vi "Main.vi"() -> ()   [LabVIEW 2018]
doc: "Cet exemple de projet Mesure continue est basé sur le modèle Gestionnaire de messages dans une file d'attente.\n\nLa boucle de gestion d'événements génère des messages en fonction des actions sur l'interface utilisateur.\n\nLa boucle de gestion de messages traite les messages générés par la boucle de gestion d'événements ou par d'autres messages. Il y a aussi des sous-VIs de boucle de gestion de messages d'acquisition et d'enregistrement, ainsi qu'une boucle de mise à jour du graphe déroulant."
uses:
  Acquisition/Acquisition.lvlib
  Logging/Logging.lvlib
  Settings/Settings.lvlib
  Acquisition/Signal Type.ctl
  Acquisition/Hardware Configuration.ctl
  Logging/Logging Configuration.ctl
  Settings/Settings.ctl
  support/User Event - Stop/User Event - Stop.lvlib
  controls/UI Data.ctl
  support/Message Queue/Message Queue.lvlib
  support/Message Queue/Enqueue Message (Single).vi
  controls/UI State.ctl
  <vilib>/ErrorRing/Error Ring.xnode
  Settings/Settings Dialog.vi
  support/Message Queue/Enqueue Message (Array).vi
  <vilib>/Utility/error.llb/Error Cluster From Error Code.vi
panel:
  in  "Panneaux":T1(tab)
  out "Therm 2":dbl(knob) scale=0.0..10.0
  out "Therm 1":dbl(knob) scale=0.0..10.0
  in  "Param status":bool
  out "Données":waveform(dbl)[](graph)
  out "État":string
  in  "Quitter":bool
  in  "Arrêter":bool
  in  "Démarrer":bool
  in  "Paramètres":bool
  # "MAPA Tech"
  # "TODO:\n\n- Valider l'enregistrement  du data\n- Faire sous-vi ordre 0\n- Faire sous-vi ordre 1"
  # "Changer tout cela pour des réservoir ou des vumètre ou jauge"
  # "MAPA Tech"
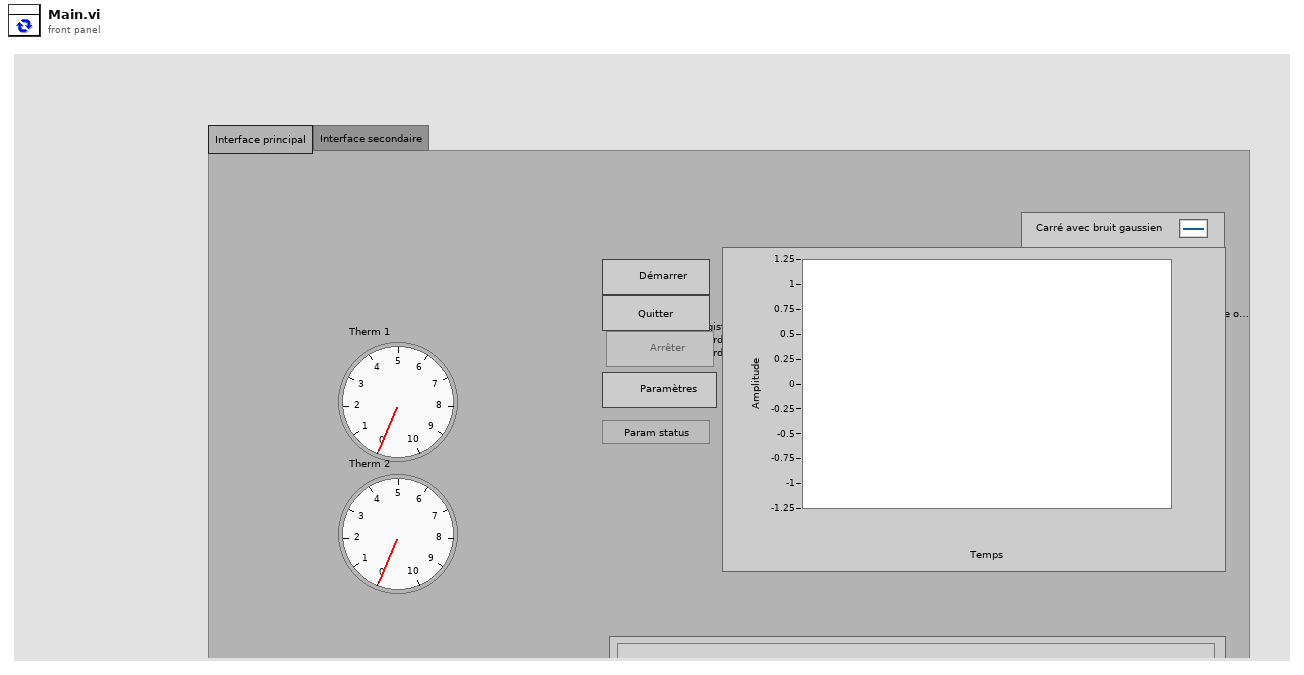
[diagram p1: front panel]
types:
  T1 = enum32{"Interface principal", "Interface secondaire"}
  T2 = typedef "UI State.ctl" = enum16{"Idle", "Acquiring and Logging", "Waiting for Exit", "Waiting for Exit (Acq Stopped)", "Waiting for Exit (Log Stopped)", "Waiting for Stop", "Waiting for Stop (Acq Stopped)", "Waiting for Stop (Log Stopped)"}
  T3 = typedef "UI Data.ctl" = cluster{"Réf. de Démarrer":refnum<vi>, "Réf. d'Arrêter":refnum<vi>, "Réf. de Paramètres":refnum<vi>, "Réf. de Quitter":refnum<vi>, "Réf. d'état":refnum<vi>, "Réf. de données":refnum<vi>, "Ref. Moyennage sélectionneur":refnum<vi>, "Ref. Param status":refnum<vi>}
  T4 = typedef "Settings.lvlib/Settings.ctl" = cluster{"Configuration du matériel":T5, "Configuration de l'enregistrement":T7}
  T5 = typedef "Acquisition.lvlib/Hardware Configuration.ctl" = cluster{"Refnum de matériel <À remplacer>":string, "Type de signal <À remplacer>":T6, "Choix de la longueur d'onde":dbl, "Nom du périphérique":tag, "Choix mode":bool}
  T6 = typedef "Acquisition.lvlib/Signal Type.ctl" = enum16{"Sine Wave", "Square with Noise", "Signal triangulaire", "Simulation DAQ"}
  T7 = typedef "Logging.lvlib/Logging Configuration.ctl" = cluster{"Chemin de base du fichier journal":path, "Référence de fichier TDMS":refnum<k34>}
  T8 = cluster{"état":bool, "code":i32, "source":string}
  T9 = typedef "Message Queue.lvlib/All Message Queues.ctl" = cluster{"IU":refnum<queue>, "Acquisition":refnum<queue>, "Enregistrement":refnum<queue>}
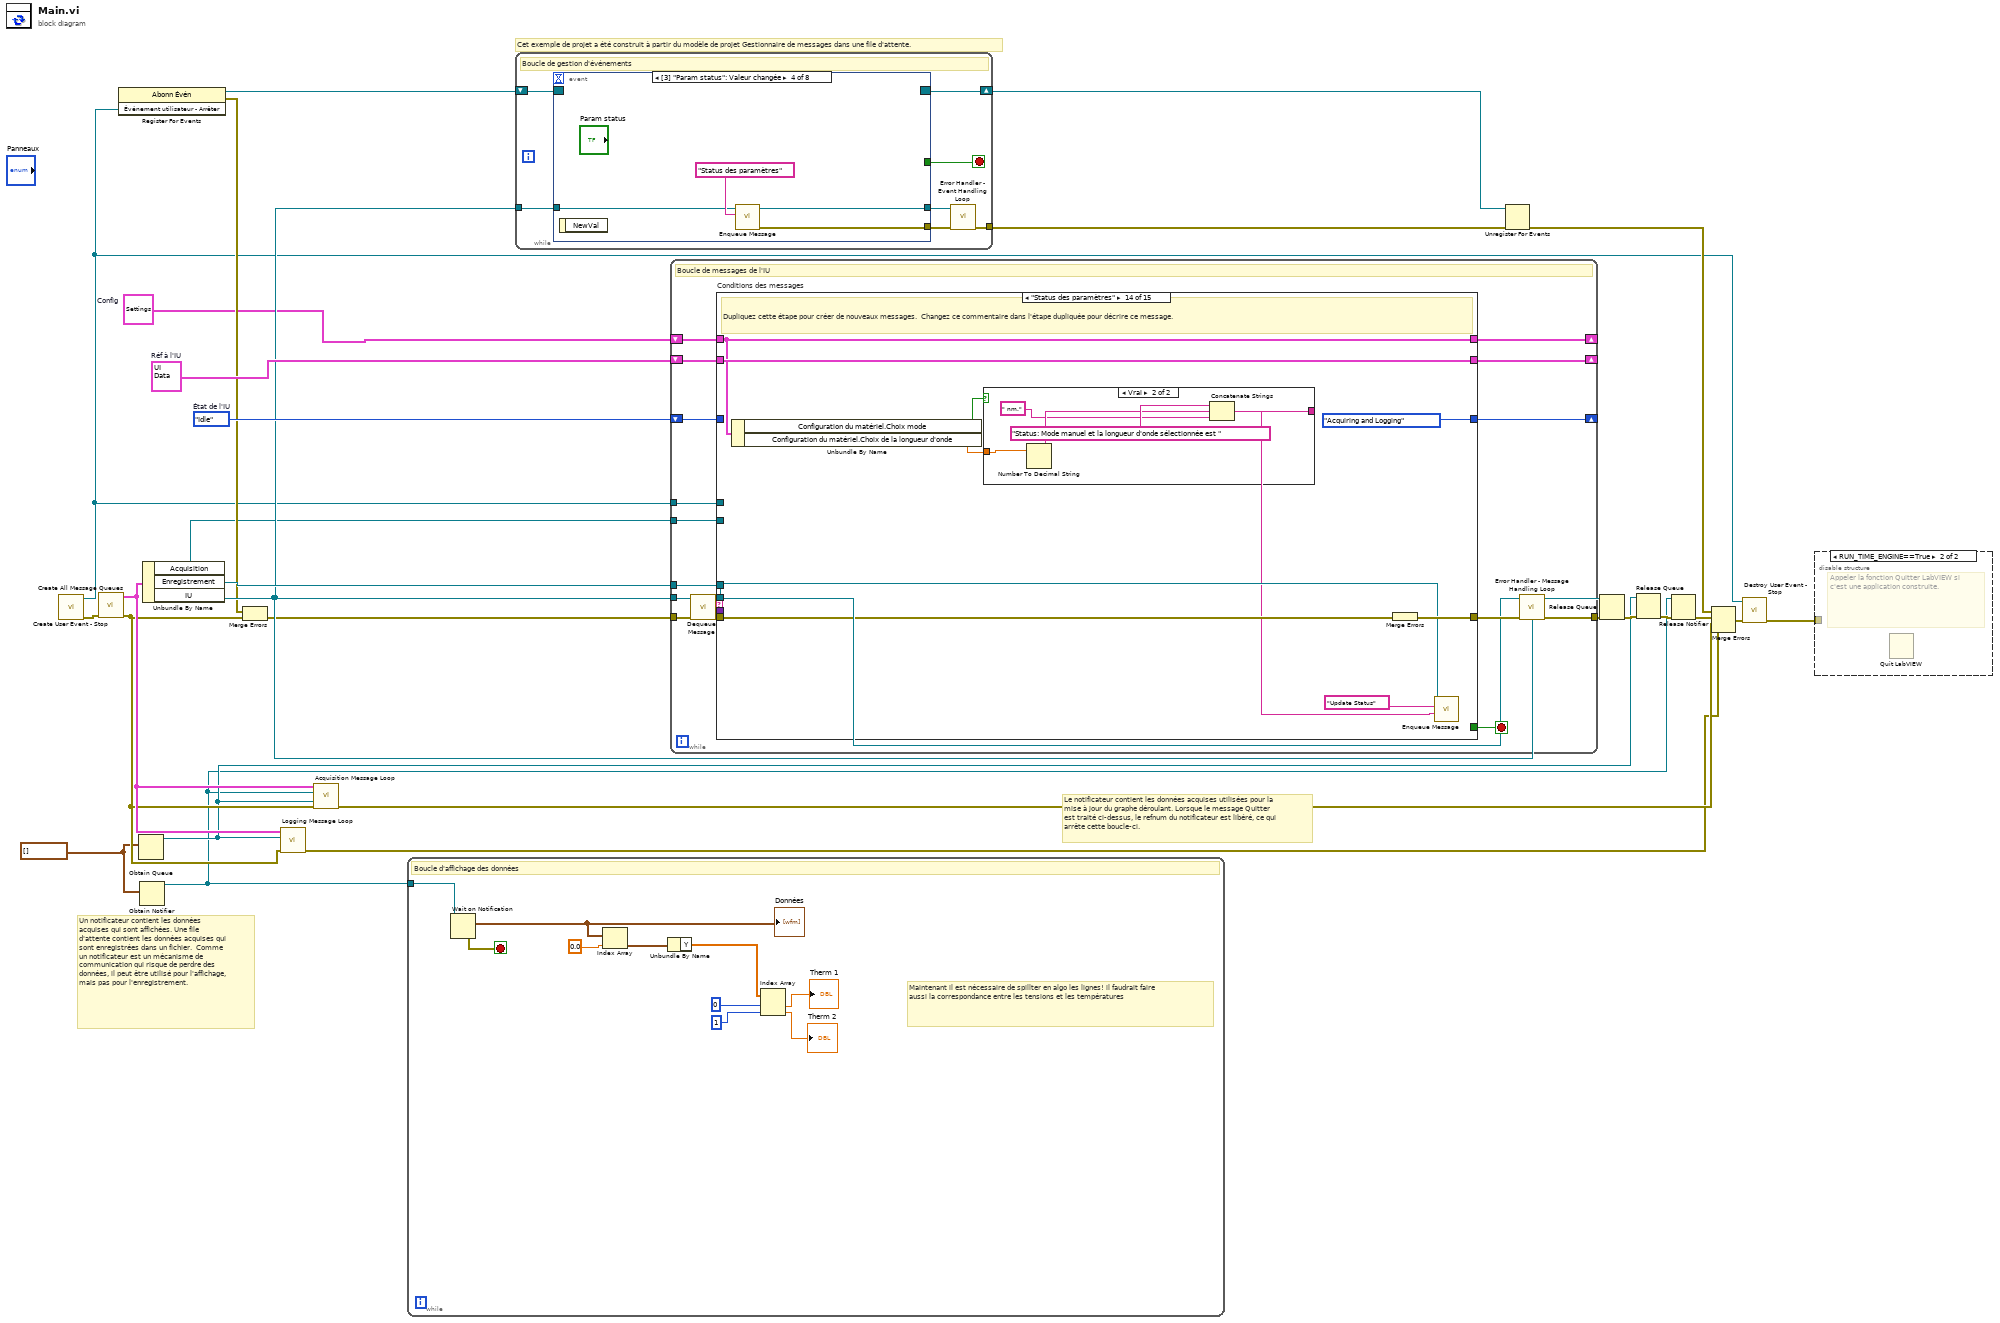
[diagram p0: block diagram]
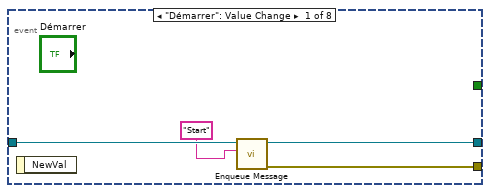
[diagram p3: hidden frame]
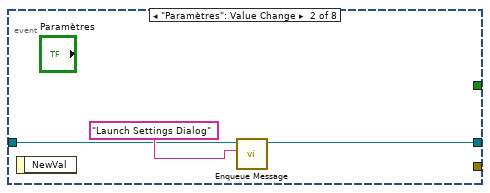
[diagram p4: hidden frame]
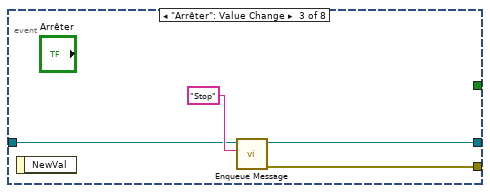
[diagram p5: hidden frame]
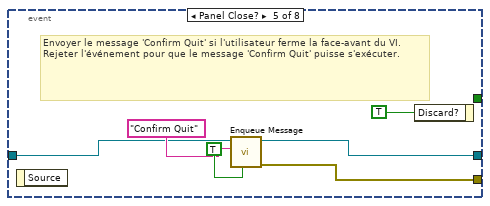
[diagram p6: hidden frame]
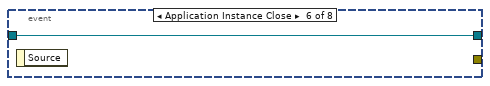
[diagram p7: hidden frame]
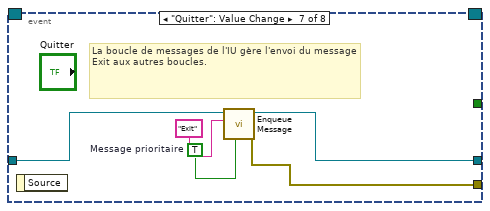
[diagram p8: hidden frame]
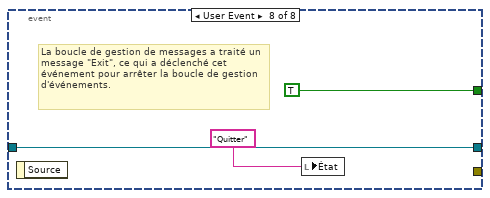
[diagram p9: hidden frame]
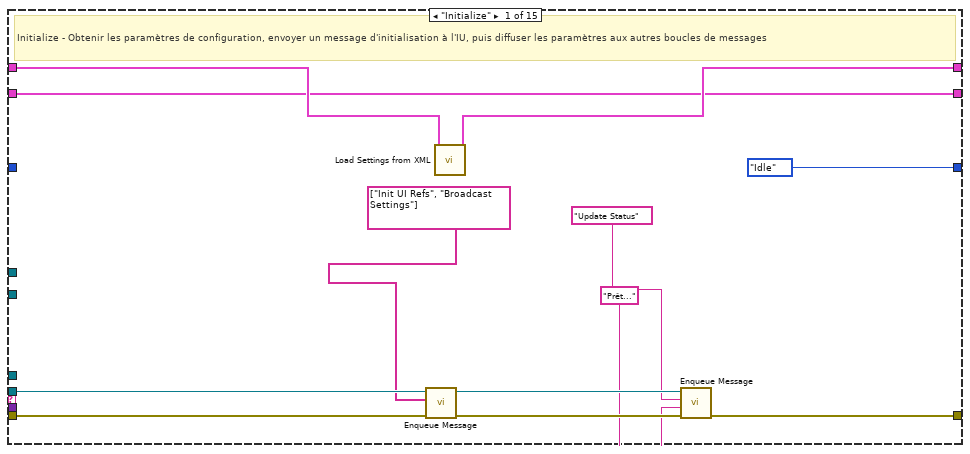
[diagram p10: hidden frame]
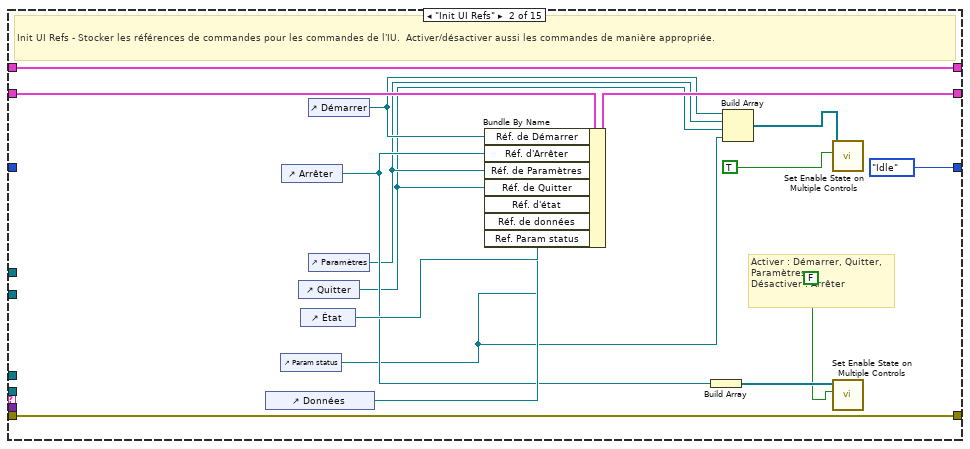
[diagram p11: hidden frame]
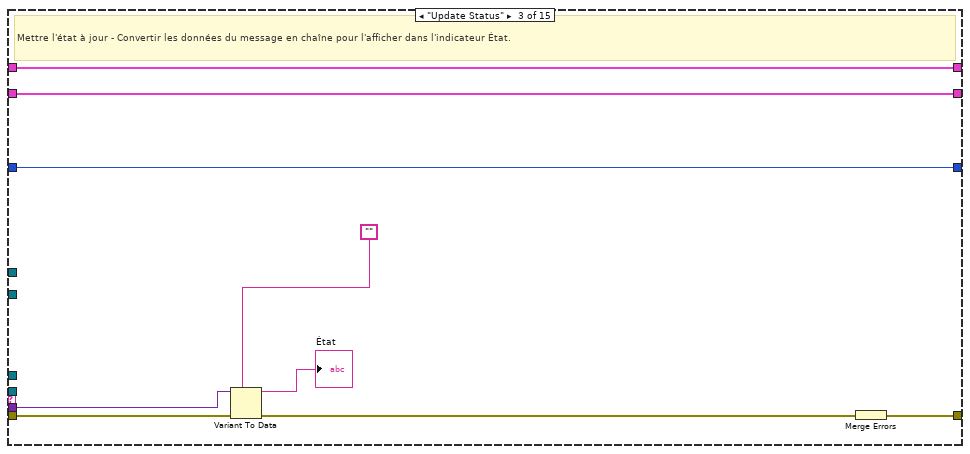
[diagram p12: hidden frame]
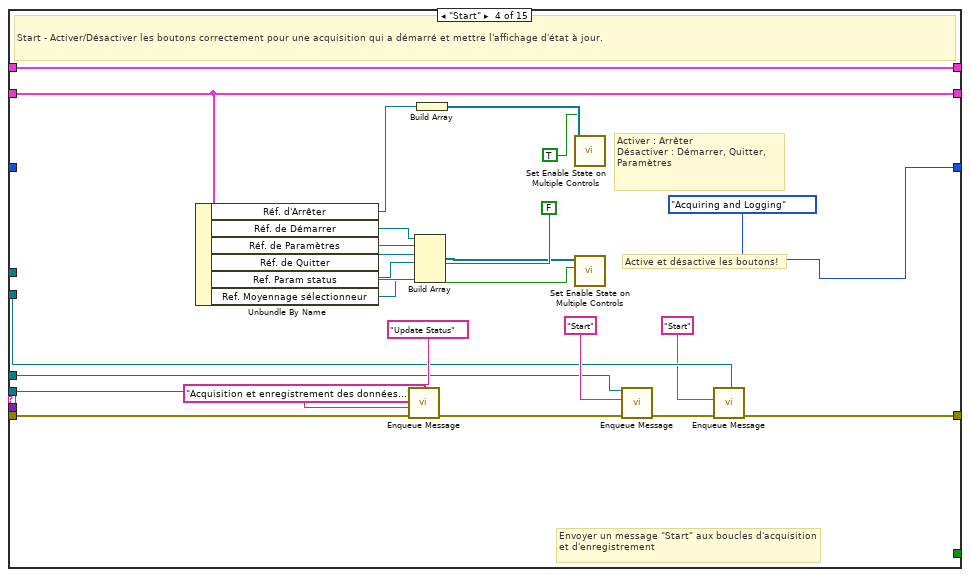
[diagram p13: hidden frame]
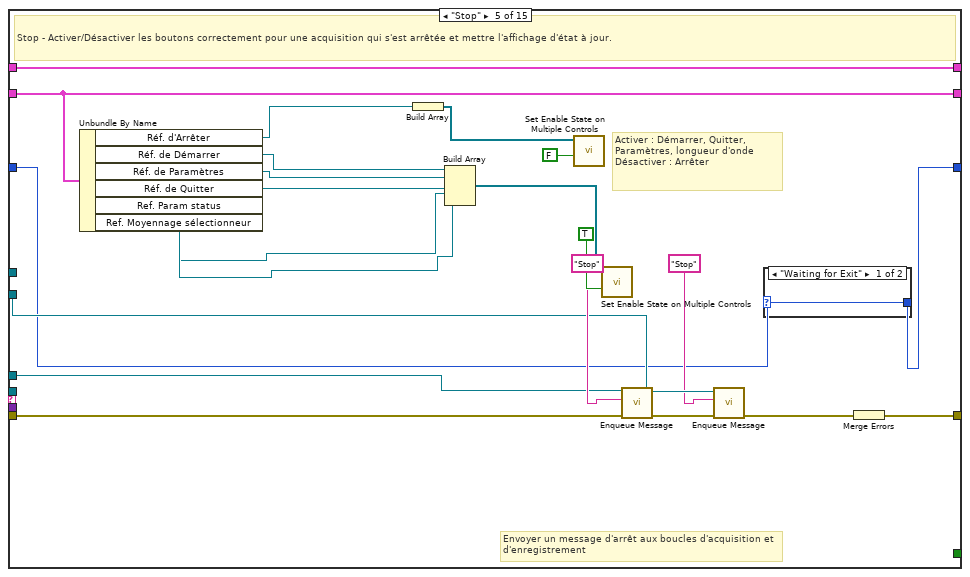
[diagram p14: hidden frame]
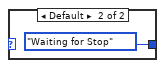
[diagram p15: hidden frame]
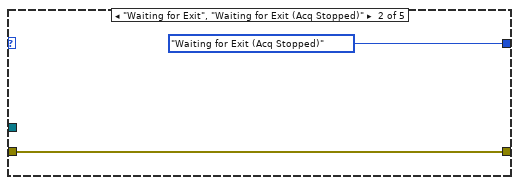
[diagram p17: hidden frame]
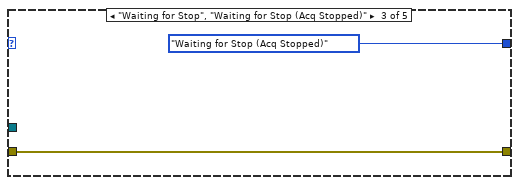
[diagram p18: hidden frame]
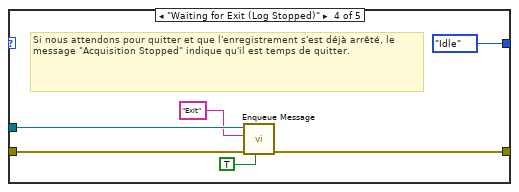
[diagram p19: hidden frame]
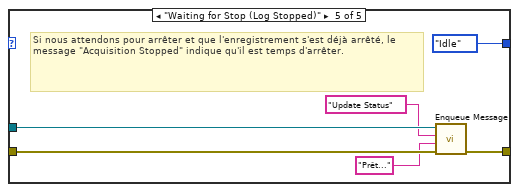
[diagram p20: hidden frame]
diagram:
  w16 = UI_State."Idle"  # État de l'IU
  w4 = waveform(dbl)[] []
  w18 = T3 {"Réf. de Démarrer"=refnum, "Réf. d'Arrêter"=refnum, "Réf. de Paramètres"=refnum, "Réf. de Quitter"=refnum, "Réf. d'état"=refnum, "Réf. de données"=refnum, "Ref. Moyennage sélectionneur"=refnum, "Ref. Param status"=refnum}  # Réf à l'IU
  w1 = T4 {"Configuration du matériel"={"Refnum de matériel <À remplacer>"="", "Type de signal <À remplacer>"=enum."Simulation DAQ", "Choix de la longueur d'onde"=500.0, "Nom du périphérique"="Dev1", "Choix mode"=FALSE}, "Configuration de l'enregistrement"={"Chemin de base du fichier journal"=path "", "Référence de fichier TDMS"=refnum}}  # Config
  # "Cet exemple de projet a été construit à partir du modèle de projet Gestionnaire de messages dans une file d'attente."
  # "Un notificateur contient les données acquises qui sont affichées. Une file d'attente contient les données acquises qui sont enregistrées dans un fichier.  Comme un notificateur est un mécanisme de communication qui risque de perdre des données, il peut être utilisé pour l'affichage, mais pas pour l'enregistrement."
  # "Le notificateur contient les données acquises utilisées pour la mise à jour du graphe déroulant. Lorsque le message Quitter est traité ci-dessus, le refnum du notificateur est libéré, ce qui arrête cette boucle-ci."
  n1 = call "Create User Event - Stop.vi"() -> ("error out"=w24:T8, "Événement utilisateur - Arrêter"=w5:refnum<user-event>)  [unwired: 10 in]
  n2 = call "Create All Message Queues.vi"("error in (no error)"=w24) -> ("error out"=w21:T8, "Files d'attente de messages en sortie"=w23:T9)  [unwired: 9 in]
  n3 = register-events(w5) -> (reference out=w9:refnum<event-registration>, error out=w7:errorcluster)  [unwired: 2 in]
  n4 = Obtain Queue(element data type=w4) -> (queue out=w3:refnum<queue>)  [unwired: 4 in, 2 out]
  n5 = Obtain Notifier(notification data type=w4) -> (notifier out=w2:refnum<notifier>)  [unwired: 3 in, 2 out]
  n6 = Unbundle By Name(w23) -> ("Acquisition"=w6:refnum<queue>, "Enregistrement"=w17:refnum<queue>, "IU"=w14:refnum<queue>)
  n7 = Merge Errors(w7, w21) -> (w8:errorcluster)
  n8 = call "Logging Message Loop.vi"("error in (no error)"=w21, "File d'attente de données"=w3, "Files d'attente de messages"=w23) -> ("error out"=w22:T8)  [unwired: 8 in]
  n9 = call "Acquisition Message Loop.vi"("Files d'attente de messages"=w23, "Notificateur de données"=w2, "File d'attente de données"=w3, "error in (no error)"=w21) -> ("error out"=w25:T8)  [unwired: 11 in]
  n10 = while "Data Display Loop" {
    tunnel: w2 -> [w36]
    stop <- w37 stop-if-true
    # "Maintenant il est nécessaire de spillter en algo les lignes! il faudrait faire aussi la correspondance entre les tensions et les températures"
    # "Boucle d'affichage des données"
    n11 = Wait on Notification(notifier=w36) -> (notification=w34:waveform(dbl)[], error out=w37:errorcluster)  [unwired: 3 in, 2 out]
    "Données" <- w34
    n12 = Index Array(array=w34, index=0.0) -> (element=w33:waveform(dbl))
    n13 = Unbundle By Name(w33) -> ("Y"=w32:dbl[])
    n14 = Index Array(array=w32, index #1=0, index #2=1) -> (element #1=→"Therm 1":dbl, element #2=→"Therm 2":dbl)
  }
  n15 = while {
    tunnel: w14 -> [w43]
    tunnel: [w40] -> w26
    shift-right: [w42] -> w19
    shift-left: w9 -> [w44]
    stop <- w41 stop-if-true
    # "Boucle de gestion d'événements"
    n16 = event shown="[3] \"Param status\": Valeur changée" {
      selector: w44 -> [_ _ _ _ _ _ _ _]
      dyn-events: [_ _ _ _ _ _ _ _] -> w42
      timeout: _ -> [_ _ _ _ _ _ _ _]
      tunnel: [_ _ _ _ _ _ _ TRUE ("Discard?")] -> w41
      tunnel: w43 -> [w48 w50 w54 w58 w63 w66 w68 w72]
      tunnel: [w46 _ w53 w57 w61 _ w71 _] -> w39
      tunnel: [w45 w49 w52 w56 w62 w66 w67 w72] -> w38
      event "Démarrer": Value Change {
        n17 = event-data() -> ()  [unwired: 1 in, 1 out]
        n18 = call-poly "Enqueue Message.vi"("Message"="Start", "File d'attente de messages"=w48) -> ("error out"=w46:T8, "File d'attente de message dup."=w45:refnum<queue>)  [unwired: 8 in]
      }
      event "Paramètres": Value Change {
        n19 = event-data() -> ()  [unwired: 1 in, 1 out]
        n20 = call-poly "Enqueue Message.vi"("Message"="Launch Settings Dialog", "File d'attente de messages"=w50) -> ("File d'attente de message dup."=w49:refnum<queue>)  [unwired: 8 in, 1 out]
      }
      event "Arrêter": Value Change {
        n21 = event-data() -> ()  [unwired: 1 in, 1 out]
        n22 = call-poly "Enqueue Message.vi"("Message"="Stop", "File d'attente de messages"=w54) -> ("error out"=w53:T8, "File d'attente de message dup."=w52:refnum<queue>)  [unwired: 8 in]
      }
      event "Param status": Value Change {
        n23 = event-data() -> ()  [unwired: 1 in, 1 out]
        n24 = call-poly "Enqueue Message.vi"("Message"="Status des paramètres", "File d'attente de messages"=w58) -> ("error out"=w57:T8, "File d'attente de message dup."=w56:refnum<queue>)  [unwired: 8 in]
      }
      event Panel Close? {
        # "Envoyer le message 'Confirm Quit' si l'utilisateur ferme la face-avant du VI. Rejeter l'événement pour que le message 'Confirm Quit' puisse s'exécuter."
        n25 = event-data() -> ()  [unwired: 1 in, 1 out]
        n26 = call-poly "Enqueue Message.vi"("Message prioritaire ? (F)"=TRUE ("Priority Message? (F)"), "Message"="Confirm Quit", "File d'attente de messages"=w63) -> ("error out"=w61:T8, "File d'attente de message dup."=w62:refnum<queue>)  [unwired: 7 in]
        n27 = event-data ("Event Filter Node")("Discard?"=TRUE) -> ()  [unwired: 1 in, 1 out]
      }
      event Application Instance Close {
        n28 = event-data() -> ()  [unwired: 1 in, 1 out]
      }
      event "Quitter": Value Change {
        w69 = TRUE  # Message prioritaire
        # "La boucle de messages de l'IU gère l'envoi du message Exit aux autres boucles."
        n29 = event-data() -> ()  [unwired: 1 in, 1 out]
        n30 = call-poly "Enqueue Message.vi"("Message prioritaire ? (F)"=w69, "Message"="Exit", "File d'attente de messages"=w68) -> ("error out"=w71:T8, "File d'attente de message dup."=w67:refnum<queue>)  [unwired: 7 in]
      }
      event User Event {
        # "La boucle de gestion de messages a traité un message \"Exit\", ce qui a déclenché cet événement pour arrêter la boucle de gestion d'événements."
        n31 = event-data() -> ()  [unwired: 1 in, 1 out]
        n32 = local write "État"("Quitter" ("Exit String")) -> ()
      }
    }
    n33 = call "Error Handler - Event Handling Loop.vi"("error in (no error)"=w39, "File d'attente de messages"=w38) -> ("erreur en entrée dup."=w40:T8)  [unwired: 8 in, 1 out]
  }
  n34 = while {
    tunnel: w14 -> [w86]
    tunnel: w5 -> [w91]
    shift-right: [w85] -> _
    shift-left: w1 -> [w84]
    shift-right: [w82] -> _
    shift-left: w18 -> [w83]
    tunnel: w6 -> [w81]
    tunnel: w17 -> [w80]
    shift-right: [w75] -> _
    shift-left: w16 -> [w76]
    tunnel: w8 -> [w90]
    tunnel: [w79] -> w27
    stop <- w92 stop-if-true
    # "Boucle de messages de l'IU"
    n35 = call "Dequeue Message.vi"("error in (no error)"=w90, "File d'attente de messages"=w86) -> ("error out"=w89:T8, "Données de message"=w87:variant, "Message"=w88:string, "File d'attente de message dup."=w77:refnum<queue>)  [unwired: 6 in]
    n36 = case "Conditions des messages" shown="\"Status des paramètres\"" w88 {
      selector: w88 -> [_ _ _ _ _ _ _ _ _ _ _ _ _ _ w330]
      tunnel: w77 -> [w96 _ _ w153 _ w180 w205 _ w245 _ w266 _ _ w317 _]
      tunnel: w89 -> [w95 w120 w128 w152 w174 w181 w206 w233 w247 w254 w265 w294 w311 w321 _]
      tunnel: [w100 w120 w129 w139 w175 w178 w203 w239 w240 w257 w264 w304 w310 w320 w329] -> w78
      tunnel: [_ _ _ _ _ _ _ _ _ _ _ TRUE _ _ _] -> w92
      tunnel: w87 -> [_ _ w127 _ _ _ _ _ _ w258 _ w292 _ _ _]
      tunnel: w91 -> [_ _ _ _ _ _ _ _ _ _ _ w305 _ _ _]
      tunnel: [w103 w119 w123 w151 w173 w184 w209 w237 w244 w262 w269 w303 w309 w315 w333] -> w85
      tunnel: w84 -> [w104 w119 w123 w151 w173 w184 w209 w237 w248 w262 w269 w303 w309 w315 w333]
      tunnel: w83 -> [w97 w118 w122 w148 w172 w183 w208 w232 w242 w261 w268 w302 w308 w319 w332]
      tunnel: [w97 w115 w122 w148 w172 w183 w208 w232 w242 w261 w268 w302 w308 w319 w332] -> w82
      tunnel: w81 -> [_ _ _ w138 w165 _ _ w231 _ _ _ w301 _ _ _]
      tunnel: w80 -> [_ _ _ w141 w168 _ _ w228 _ _ _ w300 _ _ _]
      tunnel: w76 -> [_ _ w121 _ w162 w182 w207 w230 w241 w256 w267 _ w307 _ w331]
      tunnel: [UI_State."Idle" ("UI State") UI_State."Idle" ("UI State") w121 UI_State."Acquiring and Logging" ("UI State") w163 w179 w204 w230 w241 w256 w263 UI_State."Idle" ("UI State") w307 UI_State."Acquiring and Logging" ("UI State") w331] -> w75
      frame "Initialize" {
        # "Initialize - Obtenir les paramètres de configuration, envoyer un message d'initialisation à l'IU, puis diffuser les paramètres aux autres boucles de messages"
        n37 = call-poly "Enqueue Message.vi"("error in (no error)"=w95, "Tableau de messages"=string[] ["Init UI Refs", "Broadcast Settings"], "File d'attente de messages"=w96) -> ("error out"=w102:T8, "File d'attente de message dup."=w101:refnum<queue>)  [unwired: 7 in]
        n38 = call "Load Settings from XML.vi"("Paramètres en entrée"=w104) -> ("Paramètres en sortie"=w103:T4)  [unwired: 9 in, 1 out]
        n39 = call-poly "Enqueue Message.vi"("error in (no error)"=w102, "Données de message"="Prêt..." ("Ready..."), "Message"="Update Status", "File d'attente de messages"=w101) -> ("error out"=w100:T8)  [unwired: 6 in, 1 out]
      }
      frame "Init UI Refs" {
        # "Activer : Démarrer, Quitter, Paramètres\nDésactiver : Arrêter"
        # "Init UI Refs - Stocker les références de commandes pour les commandes de l'IU.  Activer/désactiver aussi les commandes de manière appropriée."
        n40 = control-ref of="Données"() -> (w116:refnum<vi>)
        n41 = control-ref of="Param status"() -> (w105:refnum<vi>)
        n42 = control-ref of="Arrêter"() -> (w110:refnum<vi>)
        n43 = control-ref of="Quitter"() -> (w107:refnum<vi>)
        n44 = control-ref of="État"() -> (w117:refnum<vi>)
        n45 = control-ref of="Démarrer"() -> (w109:refnum<vi>)
        n46 = control-ref of="Paramètres"() -> (w108:refnum<vi>)
        n47 = Bundle By Name(cluster=w118, "Réf. de Démarrer"=w109, "Réf. d'Arrêter"=w110, "Réf. de Paramètres"=w108, "Réf. de Quitter"=w107, "Réf. d'état"=w117, "Réf. de données"=w116, "Ref. Param status"=w105) -> (w115:T3)
        n48 = Build Array(w110) -> (w112:refnum<vi>[])
        n49 = Build Array(w109, w108, w107, w105) -> (w113:refnum<vi>[])
        n50 = call "Set Enable State on Multiple Controls.vi"("Activé ?"=TRUE ("Enable?"), "Commandes"=w113) -> ()  [unwired: 10 in]
        n51 = call "Set Enable State on Multiple Controls.vi"("Activé ?"=FALSE ("Enable?"), "Commandes"=w112) -> ()  [unwired: 10 in]
      }
      frame "Update Status" {
        # "Mettre l'état à jour - Convertir les données du message en chaîne pour l'afficher dans l'indicateur État."
        n52 = Variant To Data(error in=w128, type="" ("Empty String Constant"), Variant=w127) -> (data=→"État":string, error out=w125:errorcluster)
        n53 = Merge Errors(w125) -> (w129:errorcluster)
      }
      frame "Start" {
        # "Active et désactive les boutons!"
        # "Envoyer un message \"Start\" aux boucles d'acquisition et d'enregistrement"
        # "Activer : Arrêter\nDésactiver : Démarrer, Quitter, Paramètres"
        # "Start - Activer/Désactiver les boutons correctement pour une acquisition qui a démarré et mettre l'affichage d'état à jour."
        n54 = Unbundle By Name(w148) -> ("Réf. d'Arrêter"=w130:refnum<vi>, "Réf. de Démarrer"=w131:refnum<vi>, "Réf. de Paramètres"=w132:refnum<vi>, "Réf. de Quitter"=w135:refnum<vi>, "Ref. Param status"=w134:refnum<vi>, "Ref. Moyennage sélectionneur"=w133:refnum<vi>)
        n55 = call-poly "Enqueue Message.vi"("error in (no error)"=w152, "Données de message"="Acquisition et enregistrement des données..." ("Acquiring and Logging..."), "Message"="Update Status", "File d'attente de messages"=w153) -> ("error out"=w143:T8)  [unwired: 6 in, 1 out]
        n56 = Build Array(w131, w132, w132, w135, w134, w133) -> (w146:refnum<vi>[])
        n57 = Build Array(w130) -> (w145:refnum<vi>[])
        n58 = call "Set Enable State on Multiple Controls.vi"("Activé ?"=TRUE ("Enable?"), "Commandes"=w145) -> ()  [unwired: 10 in]
        n59 = call "Set Enable State on Multiple Controls.vi"("Activé ?"=FALSE ("Enable?"), "Commandes"=w146) -> ()  [unwired: 10 in]
        n60 = call-poly "Enqueue Message.vi"("error in (no error)"=w143, "Message"="Start", "File d'attente de messages"=w141) -> ("error out"=w140:T8)  [unwired: 7 in, 1 out]
        n61 = call-poly "Enqueue Message.vi"("error in (no error)"=w140, "Message"="Start", "File d'attente de messages"=w138) -> ("error out"=w139:T8)  [unwired: 7 in, 1 out]
      }
      frame "Stop" {
        # "Envoyer un message d'arrêt aux boucles d'acquisition et d'enregistrement"
        # "Activer : Démarrer, Quitter, Paramètres, longueur d'onde\nDésactiver : Arrêter"
        # "Stop - Activer/Désactiver les boutons correctement pour une acquisition qui s'est arrêtée et mettre l'affichage d'état à jour."
        n62 = Unbundle By Name(w172) -> ("Réf. d'Arrêter"=w154:refnum<vi>, "Réf. de Démarrer"=w155:refnum<vi>, "Réf. de Paramètres"=w156:refnum<vi>, "Réf. de Quitter"=w157:refnum<vi>, "Ref. Param status"=w158:refnum<vi>, "Ref. Moyennage sélectionneur"=w159:refnum<vi>)
        n63 = Build Array(w154) -> (w160:refnum<vi>[])
        n64 = Build Array(w155, w156, w157, w158, w159) -> (w161:refnum<vi>[])
        n65 = call "Set Enable State on Multiple Controls.vi"("Activé ?"=FALSE ("Enable?"), "Commandes"=w160) -> ()  [unwired: 10 in]
        n66 = call "Set Enable State on Multiple Controls.vi"("Activé ?"=TRUE ("Enable?"), "Commandes"=w161) -> ()  [unwired: 10 in]
        n67 = call-poly "Enqueue Message.vi"("error in (no error)"=w174, "Message"="Stop", "File d'attente de messages"=w168) -> ("error out"=w167:T8)  [unwired: 7 in, 1 out]
        n68 = call-poly "Enqueue Message.vi"("error in (no error)"=w167, "Message"="Stop", "File d'attente de messages"=w165) -> ("error out"=w166:T8)  [unwired: 7 in, 1 out]
        n69 = case shown="\"Waiting for Exit\"" w162 {
          selector: w162 -> [w176 _]
          tunnel: [w176 UI_State."Waiting for Stop" ("UI State")] -> w163
          frame "Waiting for Exit" {
          }
          frame Default {
          }
        }
        n70 = Merge Errors(w166) -> (w175:errorcluster)
      }
      frame "Acquisition Stopped" {
        # "Logique déterminant quelle action entreprendre quand l'acquisition s'est arrêtée."
        n71 = case shown="Par défaut" w182 {
          selector: w182 -> [w186 _ _ _ _]
          tunnel: w181 -> [w185 w188 w190 w196 w202]
          tunnel: w180 -> [_ _ _ w194 w199]
          tunnel: [w186 UI_State."Waiting for Exit (Acq Stopped)" ("UI State") UI_State."Waiting for Stop (Acq Stopped)" ("UI State") UI_State."Idle" ("UI State") UI_State."Idle" ("UI State")] -> w179
          tunnel: [w185 w188 w190 w195 w200] -> w178
          frame Default {
          }
          frame "Waiting for Exit", "Waiting for Exit (Acq Stopped)" {
          }
          frame "Waiting for Stop", "Waiting for Stop (Acq Stopped)" {
          }
          frame "Waiting for Exit (Log Stopped)" {
            # "Si nous attendons pour quitter et que l'enregistrement s'est déjà arrêté, le message \"Acquisition Stopped\" indique qu'il est temps de quitter."
            n72 = call-poly "Enqueue Message.vi"("Message prioritaire ? (F)"=TRUE ("Priority Message? (F)"), "error in (no error)"=w196, "Message"="Exit", "File d'attente de messages"=w194) -> ("error out"=w195:T8)  [unwired: 6 in, 1 out]
          }
          frame "Waiting for Stop (Log Stopped)" {
            # "Si nous attendons pour arrêter et que l'enregistrement s'est déjà arrêté, le message \"Acquisition Stopped\" indique qu'il est temps d'arrêter."
            n73 = call-poly "Enqueue Message.vi"("error in (no error)"=w202, "Données de message"="Prêt..." ("Ready..."), "Message"="Update Status", "File d'attente de messages"=w199) -> ("error out"=w200:T8)  [unwired: 6 in, 1 out]
          }
        }
      }
      frame "Logging Stopped" {
        # "Logique déterminant quelle action entreprendre quand l'enregistrement s'est arrêté."
        n74 = case shown="\"Waiting for Stop (Acq Stopped)\"" w207 {
          selector: w207 -> [w211 _ _ _ _]
          tunnel: w206 -> [w210 w213 w215 w221 w224]
          tunnel: w205 -> [_ _ _ w219 w223]
          tunnel: [w211 UI_State."Waiting for Exit (Log Stopped)" ("UI State") UI_State."Waiting for Stop (Log Stopped)" ("UI State") UI_State."Idle" ("UI State") UI_State."Idle" ("UI State")] -> w204
          tunnel: [w210 w213 w215 w220 w222] -> w203
          frame Default {
          }
          frame "Waiting for Exit", "Waiting for Exit (Log Stopped)" {
          }
          frame "Waiting for Stop", "Waiting for Stop (Log Stopped)" {
          }
          frame "Waiting for Exit (Acq Stopped)" {
            # "Si nous attendons pour quitter et que l'acquisition s'est déjà arrêtée, le message \"Logging Stopped\" indique qu'il est temps de quitter."
            n75 = call-poly "Enqueue Message.vi"("Message prioritaire ? (F)"=TRUE ("Priority Message? (F)"), "error in (no error)"=w221, "Message"="Exit", "File d'attente de messages"=w219) -> ("error out"=w220:T8)  [unwired: 6 in, 1 out]
          }
          frame "Waiting for Stop (Acq Stopped)" {
            # "Si nous attendons pour arrêter et que l'acquisition s'est déjà arrêtée, le message \"Logging Stopped\" indique qu'il est temps d'arrêter."
            n76 = call-poly "Enqueue Message.vi"("error in (no error)"=w224, "Données de message"="Prêt..." ("Ready..."), "Message"="Update Status", "File d'attente de messages"=w223) -> ("error out"=w222:T8)  [unwired: 6 in, 1 out]
          }
        }
      }
      frame "Broadcast settings" {
        w229 = "Update Settings" ("Message")
        # "Broadcast settings - Envoyer le message 'Update Settings' aux boucles de messages d'enregistrement et d'acquisition."
        n77 = Unbundle By Name(w237) -> ("Configuration du matériel"=w236:T5, "Configuration de l'enregistrement"=w235:T7)
        n78 = call-poly "Enqueue Message.vi"("Données de message"=w236, "Message"=w229, "File d'attente de messages"=w231) -> ("error out"=w238:T8)  [unwired: 7 in, 1 out]
        n79 = call-poly "Enqueue Message.vi"("error in (no error)"=w238, "Données de message"=w235, "Message"=w229, "File d'attente de messages"=w228) -> ("error out"=w234:T8)  [unwired: 6 in, 1 out]
        n80 = Merge Errors(w234, w233) -> (w239:errorcluster)
      }
      frame "Launch Settings Dialog" {
        # "Launch Settings Dialog - Lancer la boîte de dialogue Paramètres quand l'utilisateur clique sur le bouton Paramètres."
        n81 = call-by-ref "?"("error in (no error)"=w247, "Paramètres en entrée"=w248) -> ("error out"=w243:T8, "Annulation ?"=w246:bool, "Paramètres en sortie"=w244:T4)  [unwired: 8 in, 3 out]
        n82 = case shown="Faux" w246 {
          tunnel: w245 -> [w252 _]
          tunnel: w243 -> [w251 w253]
          tunnel: [w250 w253] -> w240
          frame False {
            n83 = call-poly "Enqueue Message.vi"("error in (no error)"=w251, "Message"="Broadcast Settings", "File d'attente de messages"=w252) -> ("error out"=w250:T8)  [unwired: 7 in, 1 out]
          }
          frame True {
          }
        }
      }
      frame "Error" {
        # "Error - Afficher une boîte de dialogue d'erreur. Ce message est envoyé par les VIs \"Error Handler\" à la fin de l'exécution de chaque boucle de cette application."
        n84 = Variant To Data(error in=w254, type=errorcluster {"status"=FALSE, "code"=0, "source"=""} ("error constant"), Variant=w258) -> (data=w255:errorcluster, error out=w259:errorcluster)
        n85 = call <vilib>:"Simple Error Handler.vi"("error in (no error)"=w255) -> ()  [unwired: 4 in, 5 out]
        n86 = Merge Errors(w259) -> (w257:errorcluster)
      }
      frame "Confirm Quit" {
        # "Confirm Quit - Message qui confirme si l'utilisateur voulait vraiment quitter l'application."
        n87 = case shown="\"Acquiring and Logging\"" w267 {
          tunnel: w266 -> [w275 w279]
          tunnel: w265 -> [w274 w278]
          tunnel: [w273 w277] -> w264
          tunnel: [UI_State."Idle" ("UI State") w276] -> w263
          frame Default {
            # "Si 'Confirm Quit' survient alors que le système est inactif, le message de confirmation est inutile."
            n88 = call-poly "Enqueue Message.vi"("Message prioritaire ? (F)"=TRUE ("Priority Message? (F)"), "error in (no error)"=w274, "Message"="Exit", "File d'attente de messages"=w275) -> ("error out"=w273:T8)  [unwired: 6 in, 1 out]
          }
          frame "Acquiring and Logging" {
            n89 = Two Button Dialog(message="Voulez-vous vraiment quitter en cours d'acquisition ?" ("Confirm Quit Message"), 1:"Non" ("No"), 2:"Oui" ("Yes")) -> (T button?=w280:bool)
            n90 = case shown="Vrai" w280 {
              tunnel: w279 -> [_ w289]
              tunnel: w278 -> [w285 w290]
              tunnel: [w285 w288] -> w277
              tunnel: [UI_State."Acquiring and Logging" ("UI State") UI_State."Waiting for Exit" ("UI State")] -> w276
              frame False {
                # "L'utilisateur ne voulait pas quitter."
              }
              frame True {
                n91 = call-poly "Enqueue Message.vi"("error in (no error)"=w290, "Message"="Stop", "File d'attente de messages"=w289) -> ("error out"=w288:T8)  [unwired: 7 in, 1 out]
              }
            }
          }
        }
      }
      frame "Exit" {
        w296 = TRUE ("Priority Message? (F)")
        w297 = "Exit" ("Message")
        # "Afficher une boîte de dialogue d'erreur si 'Exit' a été appelé suite à une erreur."
        # "Arrêter le VI"
        # "Exit - Envoyer des messages Exit aux boucles d'acquisition et d'enregistrerment, et déclencher l'événement utilisateur pour arrêter la boucle de gestion d'événements."
        n92 = Variant To Data(type=errorcluster {"status"=FALSE, "code"=0, "source"=""} ("error constant"), Variant=w292) -> (data=w291:errorcluster)  [unwired: 1 in, 1 out]
        n93 = call <vilib>:"Simple Error Handler.vi"("error in (no error)"=w291) -> ()  [unwired: 4 in, 5 out]
        n94 = call-poly "Enqueue Message.vi"("Message prioritaire ? (F)"=w296, "error in (no error)"=w294, "Message"=w297, "File d'attente de messages"=w301) -> ("error out"=w298:T8)  [unwired: 6 in, 1 out]
        n95 = call-poly "Enqueue Message.vi"("Message prioritaire ? (F)"=w296, "error in (no error)"=w298, "Message"=w297, "File d'attente de messages"=w300) -> ("error out"=w295:T8)  [unwired: 6 in, 1 out]
        n96 = call "Fire User Event - Stop.vi"("error in (no error)"=w295, "Événement utilisateur - Arrêt"=w305) -> ("error out"=w304:T8)  [unwired: 9 in]
      }
      frame "---Copy This Frame---" {
        # "Dupliquez cette étape pour créer de nouveaux messages.  Changez ce commentaire dans l'étape dupliquée pour décrire ce message."
        n97 = Merge Errors(w311) -> (w310:errorcluster)
      }
      frame "Status des paramètres" {
        # "Dupliquez cette étape pour créer de nouveaux messages.  Changez ce commentaire dans l'étape dupliquée pour décrire ce message."
        n98 = Unbundle By Name(w315) -> ("Configuration du matériel.Choix mode"=w314:bool, "Configuration du matériel.Choix de la longueur d'onde"=w313:dbl)
        n99 = case shown="Vrai" w314 {
          tunnel: [w322 w327] -> w312
          tunnel: w313 -> [_ w328]
          frame False {
            n100 = Concatenate Strings ("Concaténer des chaînes")("Status: Mode automatique") -> (w322:string)
          }
          frame True {
            n101 = Number To Decimal String(number=w328) -> (decimal integer string=w325:string)  [unwired: 1 in]
            n102 = Concatenate Strings ("Concaténer des chaînes")("Status: Mode manuel et la longueur d'onde sélectionnée est ", w325, " nm.") -> (w327:string)
          }
        }
        n103 = Merge Errors(w321) -> (w320:errorcluster)
        n104 = call-poly "Enqueue Message.vi"("Données de message"=w312, "Message"="Update Status", "File d'attente de messages"=w317) -> ()  [unwired: 7 in, 2 out]
      }
      frame Default {
        # "La condition 'Par défaut' ne s'exécute que s'il y a un message qui n'est défini dans aucune des autres conditions.  Renvoyer une erreur de programmation."
        n105 = xnode ("Error Ring")("paramètre 0"=w330) -> ("sortie d'erreur"=w329:errorcluster)
      }
    }
    n106 = call "Error Handler - Message Handling Loop.vi"("error in (no error)"=w78, "File d'attente de messages"=w77) -> ("erreur en entrée dup."=w79:T8)  [unwired: 8 in, 1 out]
  }
  n107 = Unregister For Events(event registration refnum=w19, error in=w26) -> (error out=w20:errorcluster)
  n108 = Release Queue(queue=w14, error in (no error)=w27) -> (error out=w12:errorcluster)  [unwired: 1 in, 2 out]
  n109 = Release Queue(queue=w3, error in (no error)=w12) -> (error out=w11:errorcluster)  [unwired: 1 in, 2 out]
  n110 = Release Notifier(notifier=w2, error in (no error)=w11) -> (error out=w10:errorcluster)  [unwired: 1 in, 2 out]
  n111 = Merge Errors(w20, w10, w25, w22) -> (w15:errorcluster)
  n112 = call "Destroy User Event - Stop.vi"("error in (no error)"=w15, "Événement utilisateur - Arrêt"=w5) -> ("error out"=w13:T8)  [unwired: 9 in]
  n113 = disable-structure "Conditional Disable Structure" shown="RUN_TIME_ENGINE==True" {
    disable-tunnel: w13 -> [_ _]
    frame condition #0 (active) {
    }
    frame condition #1 {
      # "Appeler la fonction Quitter LabVIEW si c'est une application construite."
      n114 = Quit LabVIEW() -> ()  [unwired: 1 in]
    }
  }
